vi "autocorrelator-final version.vi"() -> ()   [LabVIEW 2011]
uses:
  <instrlib>/Generators/filename generator (number).vi
  <vilib>/Waveform/WDTOps.llb/WDT Get XY Value DBL.vi
  <vilib>/Utility/file.llb/Write To Spreadsheet File (DBL).vi
  <instrlib>/Filename Generator.lvlib
panel:
  out "Iterate Num":i32=3
  in  "Experiment Condition":string="test"
  in  "Folder":path=path "C:/Infiniium/Qifan/20150406/autocorrelation"
  in  "stop":bool
  out "XY Graph 2":cluster{sgl[], dbl[]}(graph)
  out "XY Graph-1mm correspond to 6.7ps":cluster{sgl[], dbl[]}(graph)
  in  "Scan Range (mm)":sgl=11.5
  in  "Scan Center (mm)":sgl=6.0
  in  "HWSerialNum":i32=83837638
  in  "MG17Motor":refnum<k7>(container)
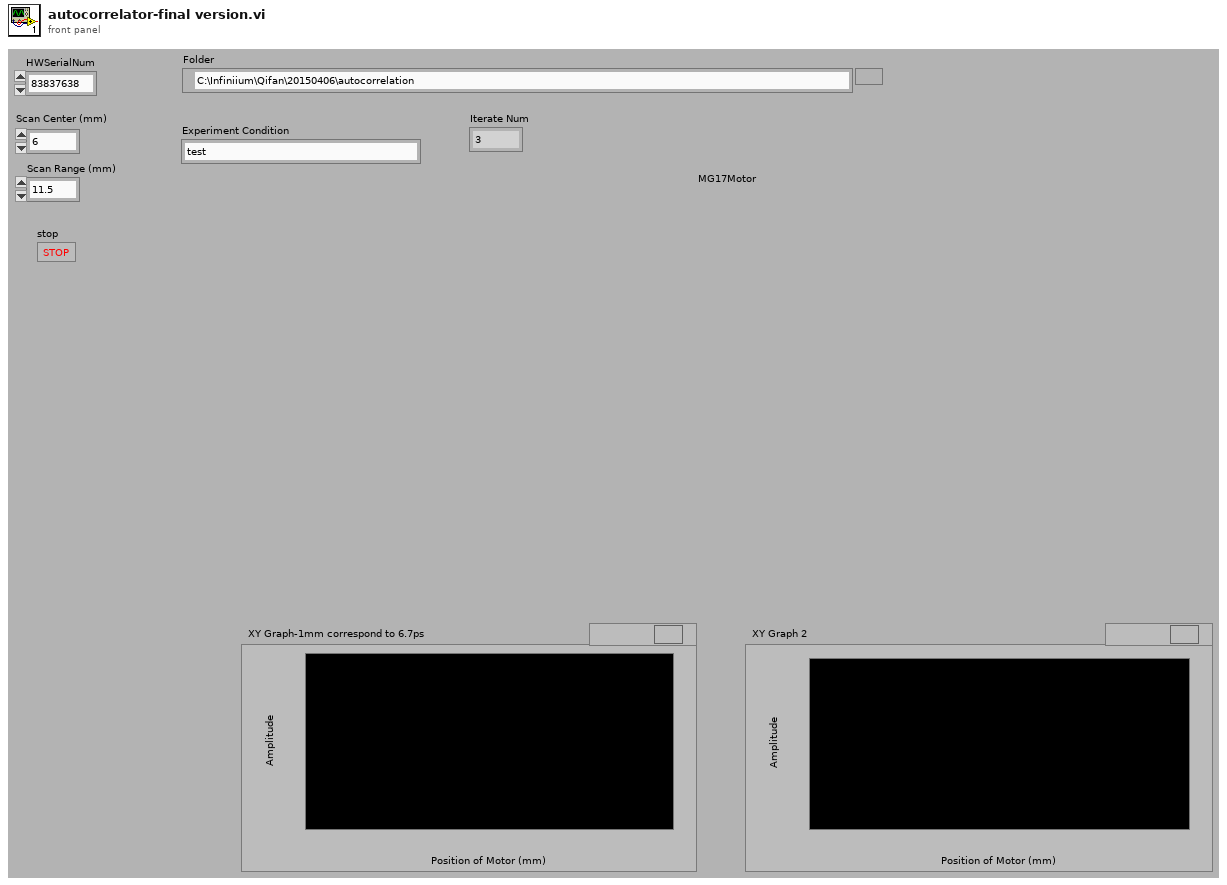
[diagram p1: front panel]
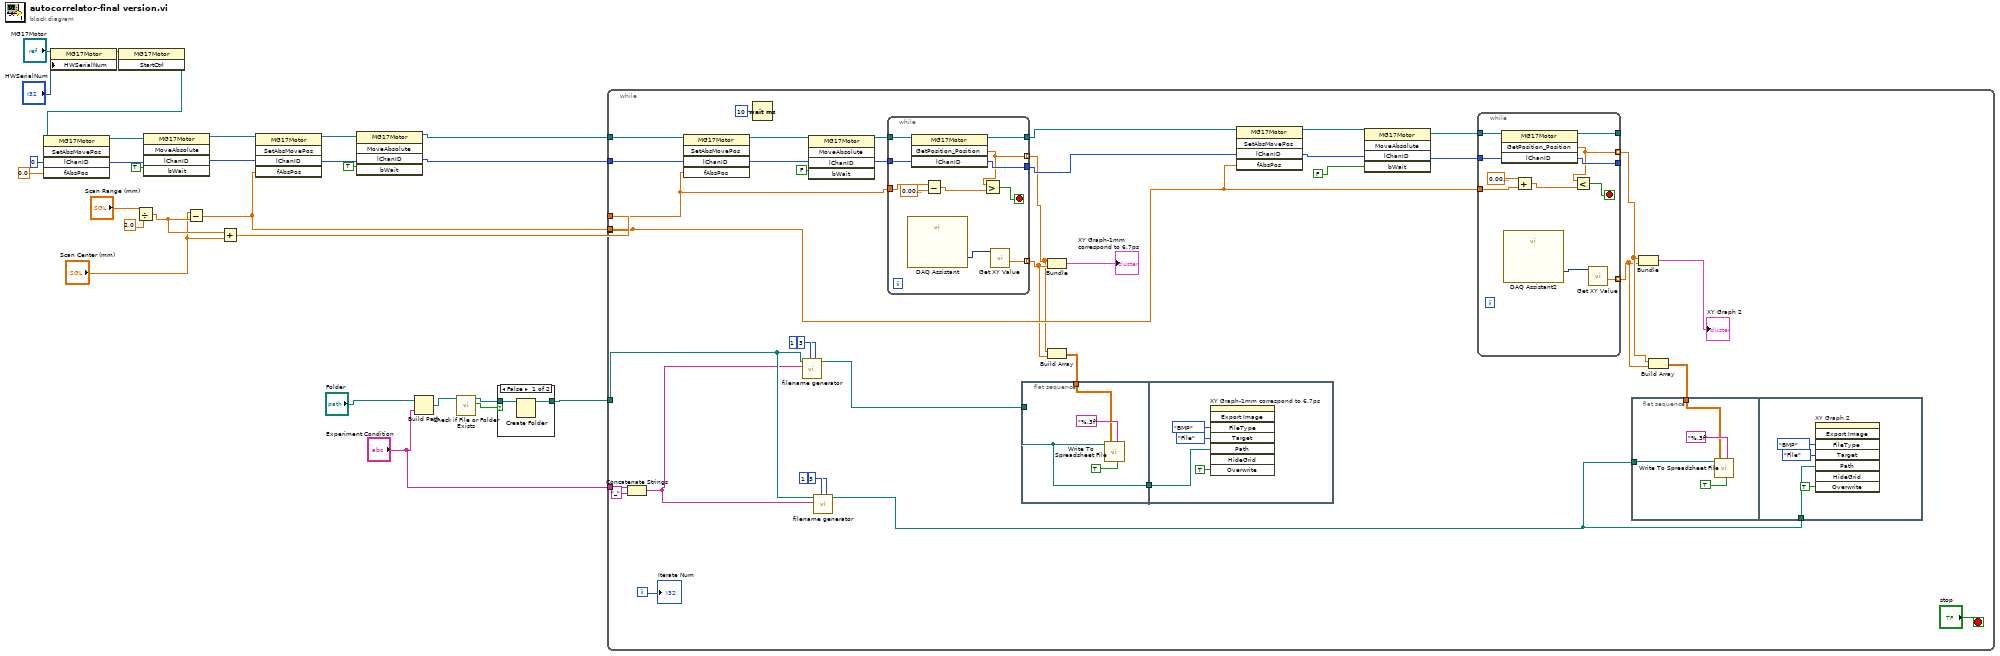
[diagram p0: block diagram]
diagram:
  n1 = property class="MG17Motor"(reference="MG17Motor", "HWSerialNum"="HWSerialNum") -> (reference out=w26:refnum<k7>)  [unwired: 1 in, 1 out]
  n2 = invoke class="MG17Motor" method="StartCtrl"(reference=w26) -> (reference out=w20:refnum<k7>)  [unwired: 2 in, 2 out]
  n3 = invoke class="MG17Motor" method="SetAbsMovePos"(reference=w20, "lChanID"=0, "fAbsPos"=sgl 0.0) -> (reference out=w25:refnum<k7>, "lChanID"=w24:i32)  [unwired: 2 in, 3 out]
  n4 = Divide(x="Scan Range (mm)", y=sgl 2.0) -> (x/y=w10:sgl)
  n5 = invoke class="MG17Motor" method="MoveAbsolute"(reference=w25, "lChanID"=w24, "bWait"=TRUE) -> (reference out=w16:refnum<k7>, "lChanID"=w15:i32)  [unwired: 2 in, 3 out]
  n6 = Subtract(x="Scan Center (mm)", y=w10) -> (x-y=w7:sgl)
  n7 = Add(x=w10, y="Scan Center (mm)") -> (x+y=w8:sgl)
  n8 = invoke class="MG17Motor" method="SetAbsMovePos"(reference=w16, "lChanID"=w15, "fAbsPos"=w7) -> (reference out=w19:refnum<k7>, "lChanID"=w18:i32)  [unwired: 2 in, 3 out]
  n9 = invoke class="MG17Motor" method="MoveAbsolute"(reference=w19, "lChanID"=w18, "bWait"=TRUE) -> (reference out=w14:refnum<k7>, "lChanID"=w13:i32)  [unwired: 2 in, 3 out]
  n10 = Build Path(base path="Folder", name or relative path="Experiment Condition") -> (appended path=w4:path)
  n11 = call <vilib>:"Check if File or Folder Exists.vi"("path"=w4) -> ("file or folder exists?"=w5:bool, "dup path"=w6:path)  [unwired: 8 in, 1 out]
  n12 = case shown="False" w5 {
    tunnel: [w30 w31] -> w3
    tunnel: w6 -> [w29 w31]
    frame False {
      n13 = Create Folder(path (use dialog)=w29) -> (created path=w30:path)  [unwired: 2 in, 2 out]
    }
    frame True {
    }
  }
  n14 = while {
    tunnel: w14 -> [w66]
    tunnel: w13 -> [w65]
    tunnel: w8 -> [w54]
    tunnel: [w51] -> _
    tunnel: w7 -> [w51]
    tunnel: w3 -> [w39]
    tunnel: "Experiment Condition" -> [w37]
    i -> [w34]
    stop <- "stop" stop-if-true
    n15 = Concatenate Strings(w37, "_" ("string")) -> (w36:string)
    n16 = invoke class="MG17Motor" method="SetAbsMovePos"(reference=w66, "lChanID"=w65, "fAbsPos"=w54) -> (reference out=w68:refnum<k7>, "lChanID"=w67:i32)  [unwired: 2 in, 3 out]
    n17 = Wait (ms)(milliseconds to wait=u32 10) -> ()  [unwired: 1 out]
    n18 = call-poly <instrlib>:"filename generator.vi"("digits (2)"=3, "start number (0)"=1, "filename root"=w36, "root folder"=w39) -> ("filename"=w44:path)  [unwired: 6 in, 1 out]
    n19 = invoke class="MG17Motor" method="MoveAbsolute"(reference=w68, "lChanID"=w67, "bWait"=FALSE) -> (reference out=w63:refnum<k7>, "lChanID"=w64:i32)  [unwired: 2 in, 3 out]
    n20 = call-poly <instrlib>:"filename generator.vi"("digits (2)"=3, "start number (0)"=1, "filename root"=w36, "root folder"=w39) -> ("filename"=w38:path)  [unwired: 6 in, 1 out]
    n21 = while {
      tunnel: w64 -> [w107]
      tunnel: w63 -> [w106]
      tunnel: [w103] -> w46 mode=indexing
      tunnel: [w105] -> w58
      tunnel: [w104] -> w57
      tunnel: w54 -> [w102]
      tunnel: [w97] -> w47 mode=indexing
      stop <- w99 stop-if-true
      n22 = call "DAQ Assistant"() -> ("data"=w98:dynamicdata)  [unwired: 17 in, 2 out]
      n23 = invoke class="MG17Motor" method="GetPosition_Position"(reference=w106, "lChanID"=w107) -> (reference out=w105:refnum<k7>, "GetPosition_Position"=w103:sgl, "lChanID"=w104:i32)  [unwired: 2 in, 1 out]
      n24 = Subtract(x=w102, y=sgl 0.01) -> (x-y=w100:sgl)
      n25 = Greater?(x=w103, y=w100) -> (0:w99:bool)
      n26 = call-poly <vilib>:"Get XY Value.vi"("waveform in"=w98) -> ("Y value"=w97:dbl)  [unwired: 6 in, 4 out]
    }
    n27 = flat-sequence {
      tunnel: w45 -> [w79]
      tunnel: w44 -> [w78]
      tunnel: [w78] -> w40
      tunnel: w40 -> [w82]
      frame #0 {
        n28 = call-poly <vilib>:"Write To Spreadsheet File.vi"("transpose? (no:F)"=TRUE, "format (%.3f)"="%.3f", "2D data"=w79, "file path (dialog if empty)"=w78) -> ()  [unwired: 4 in, 1 out]
      }
      frame #1 {
        n29 = invoke on="XY Graph-1mm correspond to 6.7ps" class="XYGraph (strict)" method="Export Image"("FileType"=enum32{"BMP", "EPS", "EMF", "PICT"}."BMP" ("File Type"), "Target"=enum32{"File", "Clipboard"}."File", "Path"=w82, "Overwrite"=TRUE ("Always Overwrite")) -> ()  [unwired: 4 in, 8 out]
      }
    }
    n30 = Bundle(w46, w47) -> (→"XY Graph-1mm correspond to 6.7ps":cluster{sgl[], dbl[]})  [unwired: 1 in]
    n31 = Build Array(w46, w47) -> (w45:dbl[][])
    n32 = invoke class="MG17Motor" method="SetAbsMovePos"(reference=w58, "lChanID"=w57, "fAbsPos"=w51) -> (reference out=w61:refnum<k7>, "lChanID"=w59:i32)  [unwired: 2 in, 3 out]
    n33 = invoke class="MG17Motor" method="MoveAbsolute"(reference=w61, "lChanID"=w59, "bWait"=FALSE) -> (reference out=w56:refnum<k7>, "lChanID"=w55:i32)  [unwired: 2 in, 3 out]
    n34 = while {
      tunnel: w55 -> [w96]
      tunnel: w56 -> [w95]
      tunnel: [w92] -> w43 mode=indexing
      tunnel: [w94] -> _
      tunnel: [w93] -> _
      tunnel: w51 -> [w88]
      tunnel: [w86] -> w42 mode=indexing
      stop <- w90 stop-if-true
      n35 = invoke class="MG17Motor" method="GetPosition_Position"(reference=w95, "lChanID"=w96) -> (reference out=w94:refnum<k7>, "GetPosition_Position"=w92:sgl, "lChanID"=w93:i32)  [unwired: 2 in, 1 out]
      n36 = call "DAQ Assistant2"() -> ("data"=w87:dynamicdata)  [unwired: 17 in, 2 out]
      n37 = Add(x=sgl 0.01 ("y"), y=w88) -> (x+y=w91:sgl)
      n38 = Less?(x=w92, y=w91) -> (x < y?=w90:bool)
      n39 = call-poly <vilib>:"Get XY Value.vi"("waveform in"=w87) -> ("Y value"=w86:dbl)  [unwired: 6 in, 4 out]
    }
    n40 = flat-sequence {
      tunnel: w41 -> [w71]
      tunnel: w38 -> [w70]
      tunnel: w38 -> [w77]
      frame #0 {
        n41 = call-poly <vilib>:"Write To Spreadsheet File.vi"("transpose? (no:F)"=TRUE, "format (%.3f)"="%.3f", "2D data"=w71, "file path (dialog if empty)"=w70) -> ()  [unwired: 4 in, 1 out]
      }
      frame #1 {
        n42 = invoke on="XY Graph 2" class="XYGraph (strict)" method="Export Image"("FileType"=enum32{"BMP", "EPS", "EMF", "PICT"}."BMP" ("File Type"), "Target"=enum32{"File", "Clipboard"}."File", "Path"=w77, "Overwrite"=TRUE ("Always Overwrite")) -> ()  [unwired: 4 in, 8 out]
      }
    }
    n43 = Bundle(w43, w42) -> (→"XY Graph 2":cluster{sgl[], dbl[]})  [unwired: 1 in]
    n44 = Build Array(w43, w42) -> (w41:dbl[][])
    "Iterate Num" <- w34
  }
